vi "Instrument Meas ACP (LTE).vi"(6 "Perform Autorange":bool=TRUE, 7 "OPC?(T)":bool=TRUE, 8 "error in":errorcluster {"code" format="%.0x"}, 10 "Timeout":u32=3000, 11 "Session In":refnum<visa-resource-name>="TCPIP0::K-N90X0A-00005.local::hislip0::INSTR") -> (0 "error out":errorcluster {"code" format="%.0x"}, 1 "Formatted Data":dbl[](array[numeric]), 2 "Power (dBm)":dbl, 3 "Session Out":refnum<visa-resource-name>)   [LabVIEW 2018]
doc: "Launches the Instrument I/O Assistant, which you can use to communicate with message-based instruments and graphically parse the response. For example you can communicate with an instrument that uses a serial, Ethernet, or GPIB interface."
panel:
  out "Data(str)":string[](array[string])
  # "Returns 32 comma-separated scalar results, in the following order.\n1. 0.0\n2. Total carrier power (dBm/Hz or dBm/MHz)\n3. 0.0\n4. Reference carrier power (dBm/Hz or dBm/MHz)\n5. Lower offset A - relative power (dB)\n6. Lower offset A - absolute power (dBm/Hz or dBm/MHz)\n7. Upper offset A - relative power (dB)\n8. Upper offset A - absolute power (dBm/Hz or dBm/MHz)\n9. Lower offset B - relative power (dB)\n10. Lower offset B - absolute power (dBm/Hz or dBm/MHz)\n11. Upper offset B - relative power (dB)\n12. Upper offset B - absolute power (dBm/Hz or dBm/MHz)\n...\n25. Lower offset F - relative power (dB)\n26. Lower offset F - absolute power (dBm/Hz or dBm/MHz)\n27. Upper offset F - relative power (dB)\n28. Upper offset F - absolute power (dBm/Hz or dBm/MHz)\n29. –999.0\n30. –999.0\n31. –999.0\n32. –999.0\nThe last four (29, 30, 31 and 32) results always returned –999.0.\nIf the results are not available, –999.0 is returned."
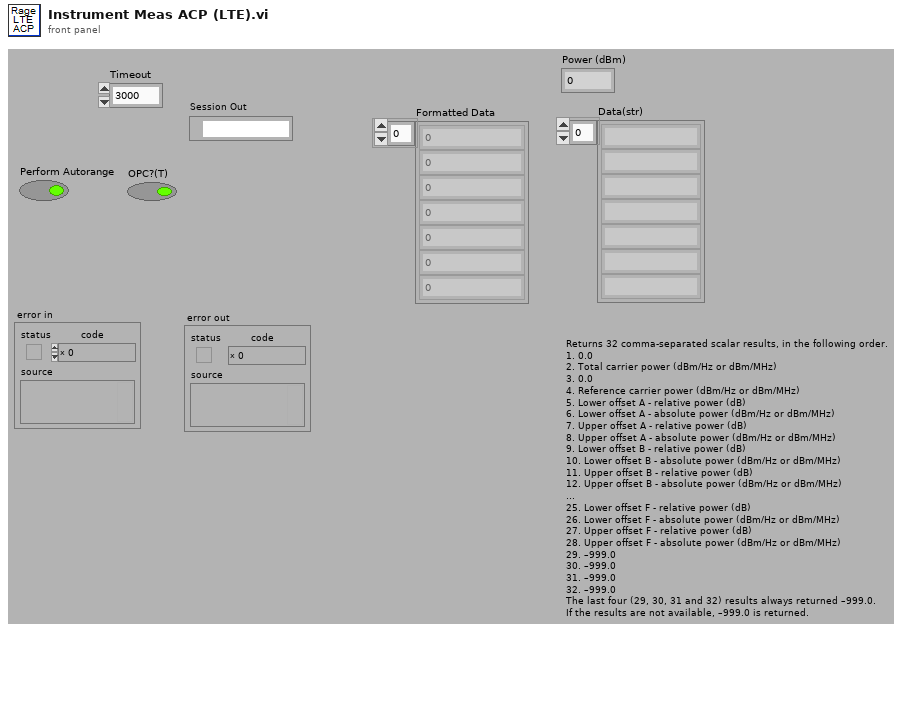
[diagram p1: front panel]
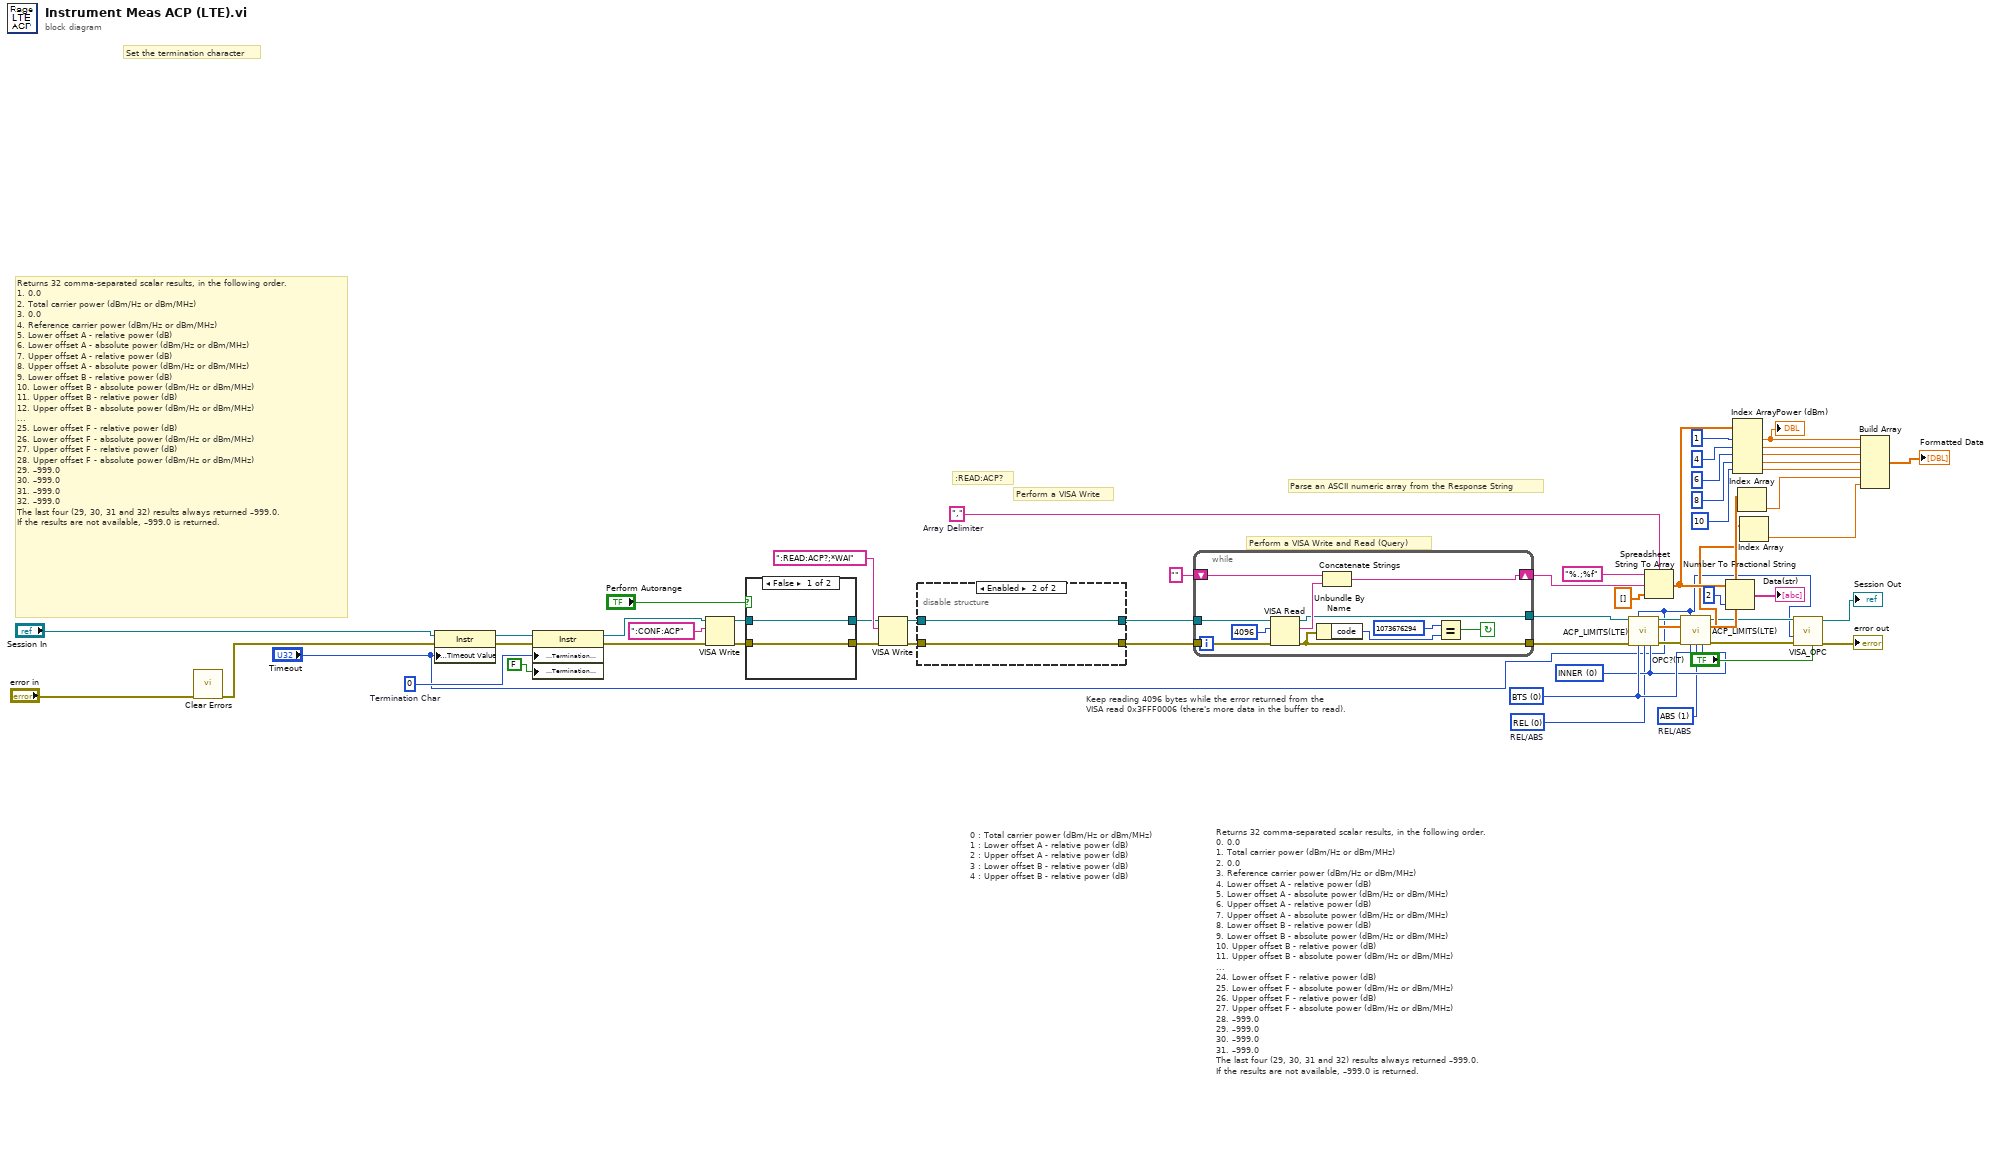
[diagram p0: block diagram]
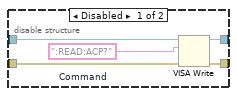
[diagram p2: hidden frame]
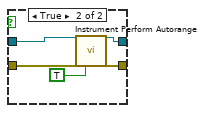
[diagram p3: hidden frame]
diagram:
  w4 = 1 items=["ABS"=1, "REL"=0]  # REL/ABS
  w5 = 0 items=["ABS"=1, "REL"=0]  # REL/ABS
  w6 = 0 items=["OUTER"=1, "INNER"=0] ("line index")
  w7 = 0 items=["MS"=1, "BTS"=0] ("BTS/MS")
  w44 = ","  # Array Delimiter
  w53 = u8 0  # Termination Char
  # ":READ:ACP?"
  # "0 : Total carrier power (dBm/Hz or dBm/MHz)\n1 : Lower offset A - relative power (dB)\n2 : Upper offset A - relative power (dB)\n3 : Lower offset B - relative power (dB)\n4 : Upper offset B - relative power (dB)"
  # "Returns 32 comma-separated scalar results, in the following order.\n0. 0.0\n1. Total carrier power (dBm/Hz or dBm/MHz)\n2. 0.0\n3. Reference carrier power (dBm/Hz or dBm/MHz)\n4. Lower offset A - relative power (dB)\n5. Lower offset A - absolute power (dBm/Hz or dBm/MHz)\n6. Upper offset A - relative power (dB)\n7. Upper offset A - absolute power (dBm/Hz or dBm/MHz)\n8. Lower offset B - relative power (dB)\n9. Lower offset B - absolute power (dBm/Hz or dBm/MHz)\n10. Upper offset B - relative power (dB)\n11. Upper offset B - absolute power (dBm/Hz or dBm/MHz)\n...\n24. Lower offset F - relative power (dB)\n25. Lower offset F - absolute power (dBm/Hz or dBm/MHz)\n26. Upper offset F - relative power (dB)\n27. Upper offset F - absolute power (dBm/Hz or dBm/MHz)\n28. –999.0\n29. –999.0\n30. –999.0\n31. –999.0\nThe last four (29, 30, 31 and 32) results always returned –999.0.\nIf the results are not available, –999.0 is returned."
  # "Returns 32 comma-separated scalar results, in the following order.\n1. 0.0\n2. Total carrier power (dBm/Hz or dBm/MHz)\n3. 0.0\n4. Reference carrier power (dBm/Hz or dBm/MHz)\n5. Lower offset A - relative power (dB)\n6. Lower offset A - absolute power (dBm/Hz or dBm/MHz)\n7. Upper offset A - relative power (dB)\n8. Upper offset A - absolute power (dBm/Hz or dBm/MHz)\n9. Lower offset B - relative power (dB)\n10. Lower offset B - absolute power (dBm/Hz or dBm/MHz)\n11. Upper offset B - relative power (dB)\n12. Upper offset B - absolute power (dBm/Hz or dBm/MHz)\n...\n25. Lower offset F - relative power (dB)\n26. Lower offset F - absolute power (dBm/Hz or dBm/MHz)\n27. Upper offset F - relative power (dB)\n28. Upper offset F - absolute power (dBm/Hz or dBm/MHz)\n29. –999.0\n30. –999.0\n31. –999.0\n32. –999.0\nThe last four (29, 30, 31 and 32) results always returned –999.0.\nIf the results are not available, –999.0 is returned."
  # "Parse an ASCII numeric array from the Response String"
  # "Perform a VISA Write and Read (Query)"
  # "Keep reading 4096 bytes while the error returned from the\nVISA read 0x3FFF0006 (there's more data in the buffer to read)."
  # "Perform a VISA Write"
  # "Set the termination character"
  n1 = call <vilib>:"Clear Errors.vi"("error in (no error)"="error in") -> ("error out"=w1:errorcluster)  [unwired: 5 in, 1 out]
  n2 = property class="Instr"(reference="Session In", error in=w1, "General Settings:Timeout Value"="Timeout") -> (reference out=w52:refnum<visa-resource-name>, error out=w55:errorcluster)
  n3 = property class="Instr"(reference=w52, error in=w55, "Message Based Settings:Termination Character"=w53, "Message Based Settings:Termination Character Enable"=FALSE ("enable")) -> (reference out=w38:refnum<visa-resource-name>, error out=w54:errorcluster)
  n4 = VISA Write(VISA resource name=w38, write buffer=":CONF:ACP", error in (no error)=w54) -> (VISA resource name out=w26:refnum<visa-resource-name>, error out=w25:errorcluster)  [unwired: 1 out]
  n5 = case shown="False" "Perform Autorange" {
    tunnel: w26 -> [w58 w64]
    tunnel: w25 -> [w59 w63]
    tunnel: [w59 w62] -> w24
    tunnel: [w58 w61] -> w23
    frame False {
    }
    frame True {
      n6 = call "Instrument Perform Autorange.vi"("Session In"=w64, "error in"=w63, "Perform AutoRange"=TRUE) -> ("Session Out"=w61:refnum<visa-resource-name>, "error out"=w62:errorcluster)  [unwired: 23 in]
    }
  }
  n7 = VISA Write(VISA resource name=w23, write buffer=":READ:ACP?;*WAI" ("StaticText"), error in (no error)=w24) -> (VISA resource name out=w37:refnum<visa-resource-name>, error out=w42:errorcluster)  [unwired: 1 out]
  n8 = disable-structure shown="Enabled" {
    disable-tunnel: [w69 w71] -> w49
    disable-tunnel: [w68 w70] -> w48
    disable-tunnel: w42 -> [w66 w70]
    disable-tunnel: w37 -> [w65 w71]
    frame Disabled {
      w67 = ":READ:ACP?"  # Command
      n9 = VISA Write(VISA resource name=w65, write buffer=w67, error in (no error)=w66) -> (VISA resource name out=w69:refnum<visa-resource-name>, error out=w68:errorcluster)  [unwired: 1 out]
    }
    frame Enabled {
    }
  }
  n10 = while {
    tunnel: w49 -> [w79]
    shift-right: [w73] -> w43
    shift-left: "" -> [w78]
    tunnel: w48 -> [w76]
    tunnel: [w75] -> w19
    tunnel: [w72] -> w20
    stop <- w74 continue-if-true
    n11 = VISA Read(VISA resource name=w79, byte count=u32 4096 ("byte count (0)"), error in (no error)=w76) -> (VISA resource name out=w72:refnum<visa-resource-name>, read buffer=w77:string, error out=w75:errorcluster)  [unwired: 1 out]
    n12 = Unbundle By Name(w75) -> ("code"=w81:i32)
    n13 = Concatenate Strings(w78, w77) -> (w73:string)
    n14 = Equal?(x=1073676294, y=w81) -> (x = y?=w74:bool)
  }
  n15 = call "ACP_LIMITS(LTE).vi"("Session In"=w20, "Timeout"="Timeout", "error in"=w19, "BTS/MS"=w7, "REL/ABS"=w5, "INNER/OUTER"=w6) -> ("Session Out"=w10:refnum<visa-resource-name>, "Limits"=w18:dbl[], "error out"=w11:errorcluster)  [unwired: 7 in]
  n16 = Spreadsheet String To Array(delimiter (Tab)=w44, format string="%.;%f", spreadsheet string=w43, array type (2D Dbl)=dbl[] []) -> (array=w21:dbl[])
  n17 = call "ACP_LIMITS(LTE).vi"("Session In"=w10, "Timeout"="Timeout", "error in"=w11, "BTS/MS"=w7, "REL/ABS"=w4, "INNER/OUTER"=w6) -> ("Session Out"=w3:refnum<visa-resource-name>, "Limits"=w9:dbl[], "error out"=w12:errorcluster)  [unwired: 7 in]
  n18 = Number To Fractional String(number=w21, precision (6)=i16 2) -> (F-format string=→"Data(str)":string[])  [unwired: 2 in]
  n19 = Index Array(array=w21, index #1=1 ("index"), index #2=4 ("index"), index #3=6 ("index"), index #4=8 ("index"), index #5=10 ("index")) -> (element #1=w16:dbl, element #2=w36:dbl, element #3=w35:dbl, element #4=w34:dbl, element #5=w33:dbl)
  "Power (dBm)" <- w16
  n20 = Index Array(array=w18) -> (element=w17:dbl)  [unwired: 1 in]
  n21 = Index Array(array=w9) -> (element=w8:dbl)  [unwired: 1 in]
  n22 = call "VISA_OPC.vi"("OPC(T)"="OPC?(T)", "error in"=w12, "Timeout"="Timeout", "Session In"=w3) -> ("error out"=→"error out":errorcluster, "Session Out"=→"Session Out":refnum<visa-resource-name>)  [unwired: 5 in, 1 out]
  n23 = Build Array(w16, w36, w35, w34, w33, w17, w8) -> (→"Formatted Data":dbl[])
